vi "SendMessageToOEP.vi"(8 "error in":errorcluster, 10 "message":string, 11 "port":u16=5556) -> (0 "error out":errorcluster)   [LabVIEW 2017]
uses:
  <vilib>/addons/zeromq/socket_type.ctl
  <vilib>/addons/zeromq/zmq_context.lvclass
  <vilib>/addons/zeromq/zeromq.lvlib
  <vilib>/addons/zeromq/zmq_socket.lvclass
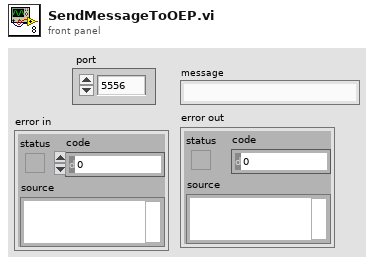
[diagram p1: front panel]
types:
  T1 = typedef "zeromq.lvlib/socket_type.ctl" = enum8{"ZMQ_PAIR", "ZMQ_PUB", "ZMQ_SUB", "ZMQ_REQ", "ZMQ_REP", "ZMQ_DEALER", "ZMQ_ROUTER", "ZMQ_PULL", "ZMQ_PUSH", "ZMQ_XPUB", "ZMQ_XSUB"}
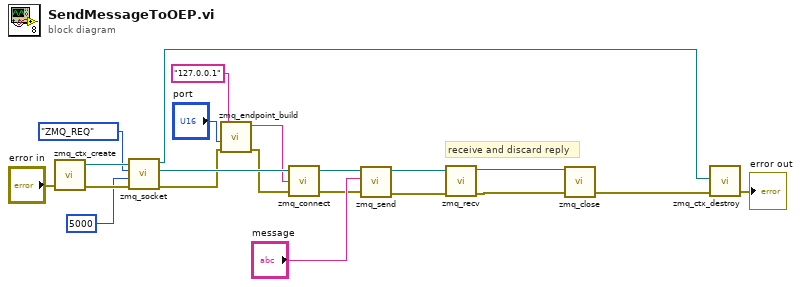
[diagram p0: block diagram]
diagram:
  # "receive and discard reply"
  n1 = call <vilib>:"zmq_ctx_create.vi"("error in"="error in") -> ("error out"=w21:errorcluster, "context out"=w20:refnum<class "zmq_context.lvclass">)  [unwired: 3 in]
  n2 = call <vilib>:"zmq_socket.vi"("error in"=w21, "linger (ms)"=5000, "socket type"=socket_type."ZMQ_REQ", "context in"=w20) -> ("error out"=w14:errorcluster, "socket out"=w17:refnum<class "zmq_socket.lvclass">, "context out"=w16:refnum<class "zmq_context.lvclass">)  [unwired: 1 in]
  n3 = call <vilib>:"zmq_endpoint_build.vi"("error in"=w14, "port"="port", "address"="127.0.0.1") -> ("error out"=w13:errorcluster, "endpoint"=w12:string)  [unwired: 2 in, 1 out]
  n4 = call <vilib>:"zmq_connect.vi"("error in"=w13, "endpoint"=w12, "socket in"=w17) -> ("error out"=w9:errorcluster, "socket out"=w10:refnum<class "zmq_socket.lvclass">)  [unwired: 1 in]
  n5 = call <vilib>:"zmq_send.vi"("error in"=w9, "data"="message", "socket in"=w10) -> ("error out"=w8:errorcluster, "socket out"=w7:refnum<class "zmq_socket.lvclass">)  [unwired: 4 in]
  n6 = call <vilib>:"zmq_recv.vi"("error in"=w8, "socket in"=w7) -> ("error out"=w6:errorcluster, "socket out"=w5:refnum<class "zmq_socket.lvclass">)  [unwired: 3 in, 3 out]
  n7 = call <vilib>:"zmq_close.vi"("error in"=w6, "socket"=w5) -> ("error out"=w4:errorcluster)  [unwired: 3 in]
  n8 = call <vilib>:"zmq_ctx_destroy.vi"("error in"=w4, "context in"=w16) -> ("error out"=→"error out":errorcluster)  [unwired: 3 in]
